vi "createClassAttribute.vi"(8 "error in (no error)":errorcluster, 10 "LVClass In":variant, 11 "WriteAttribute In":refnum<class "XMLAttributeGenerator.lvclass">) -> (0 "error out":errorcluster, 2 "AttributeString":string, 3 "WriteAttribute Out":refnum<class "XMLAttributeGenerator.lvclass">)   [LabVIEW 2014, in "XML.lvlib" / "XMLAttributeGenerator.lvclass"]
doc: "This method creates a class namespace (fully qualified string) attribute for XML generation based on the input object."
uses:
  <userlib>/Common/XML/XMLAttributeGenerator/XMLAttributeGenerator.lvclass
  <userlib>/Common/XML/XMLAttributeGenerator/AttributeElementToString.vi
  <userlib>/Common/XML/XMLAttributeGenerator/formatAttributeString.vi
  <vilib>/dlg_ctls.llb/Space Constant.vi
  <vilib>/Utility/VariantDataType/VariantType.lvlib
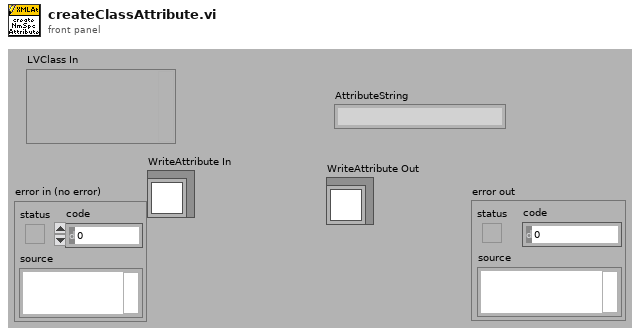
[diagram p1: front panel]
types:
  T1 = typedef "XML.lvlib/AttributeElements.ctl" = cluster{"attributeType":string, "attributeValue":string}
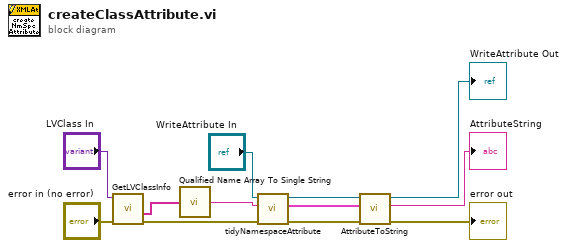
[diagram p0: block diagram]
diagram:
  n1 = call <vilib>:"GetLVClassInfo.vi"("error in (no error)"="error in (no error)", "Variant"="LVClass In") -> ("error out"=w9:errorcluster, "Fully Qualified LV Class Name"=w11:string[])  [unwired: 7 in, 1 out]
  n2 = call <vilib>:"Qualified Name Array To Single String.vi"("Fully Qualified Array"=w11) -> ("Fully Qualified String"=w8:string)
  n3 = call <userlib>:"tidyNamespaceAttribute.vi"("error in (no error)"=w9, "Fully Qualified String"=w8, "AttributeWriter In"="WriteAttribute In") -> ("error out"=w2:errorcluster, "attributeData"=w6:T1, "AttributeWriter Out"=w3:refnum<class "XMLAttributeGenerator.lvclass">)  [unwired: 6 in]
  n4 = call-poly <userlib>:"AttributeToString.vi"("error in (no error)"=w2, "attributeElement"=w6, "WriteAttribute in"=w3) -> ("error out"=→"error out":errorcluster, "AttributeString"=→"AttributeString":string, "WriteAttribute out"=→"WriteAttribute Out":refnum<class "XMLAttributeGenerator.lvclass">)  [unwired: 6 in]
